vi "VFP Network Set Binding Attributes.vi"(9 "Access Type Strings":string[](array[string]), 10 "Ctl Ref Cluster":T2, 11 "attributes":T1) -> (3 "attributes out":T1)   [LabVIEW 2016]
uses:
  <resource>/dialog/variable/SCT Attributes.ctl
  <resource>/dialog/variable/FeaturePacks/Network/VFP Network ControlRef.ctl
  <resource>/dialog/variable/FeaturePacks/Utility/VFP Util Fetch Bool Control.vi
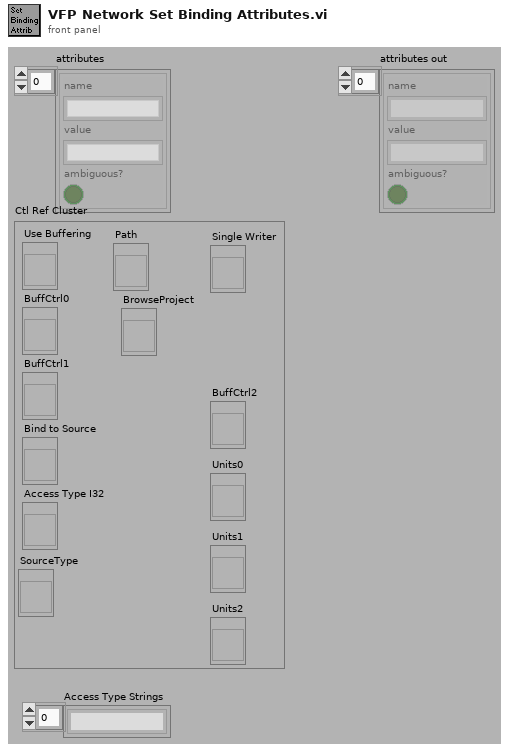
[diagram p1: front panel]
types:
  T1 = typedef "SCT Attributes.ctl" = cluster{"name":string, "value":string, "ambiguous?":bool}[]
  T2 = typedef "VFP Network ControlRef.ctl" = cluster{"Use Buffering":refnum<vi>, "BuffCtrl0":refnum<vi>, "BuffCtrl1":refnum<vi>, "Bind to Source":refnum<vi>, "Access Type I32":refnum<vi>, "Path":refnum<vi>, "BrowseProject":refnum<vi>, "Single Writer":refnum<vi>, "BuffCtrl2":refnum<vi>, "Units0":refnum<vi>, "Units1":refnum<vi>, "Units2":refnum<vi>, "SourceType":refnum<vi>}
  T3 = cluster{"name":string, "value":string, "ambiguous?":bool}
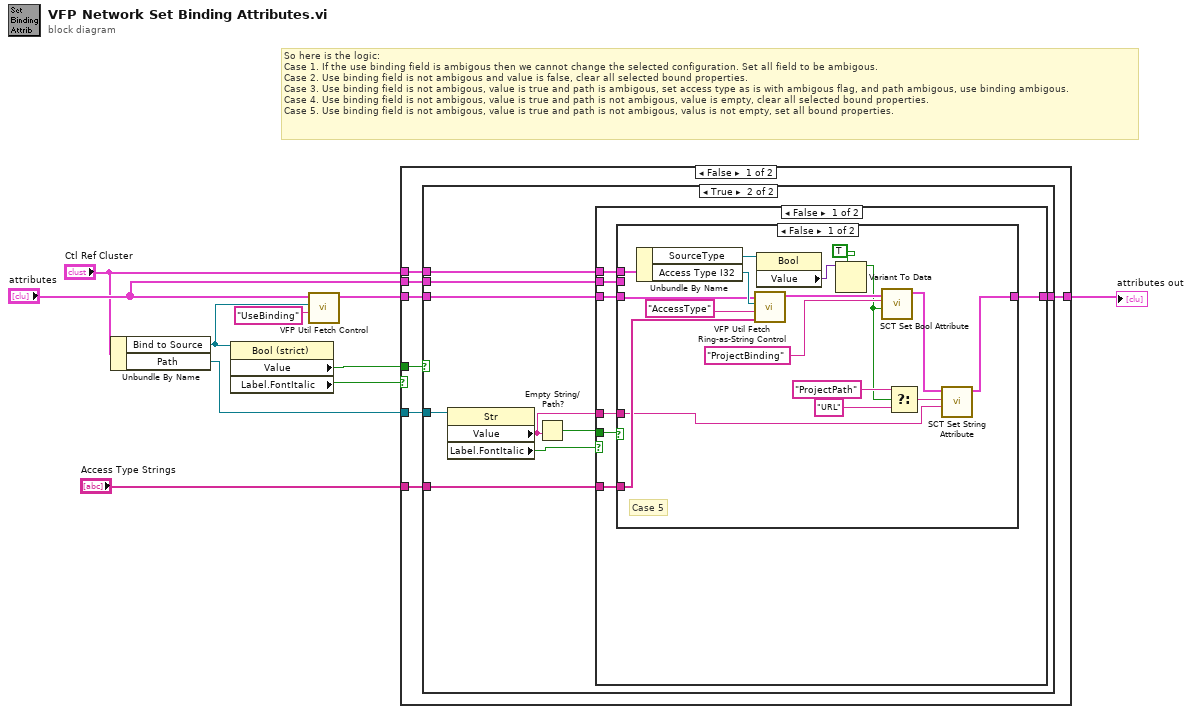
[diagram p0: block diagram]
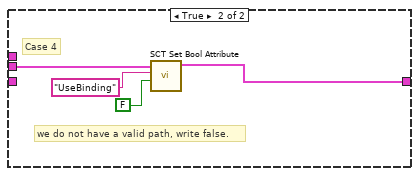
[diagram p3: hidden frame]
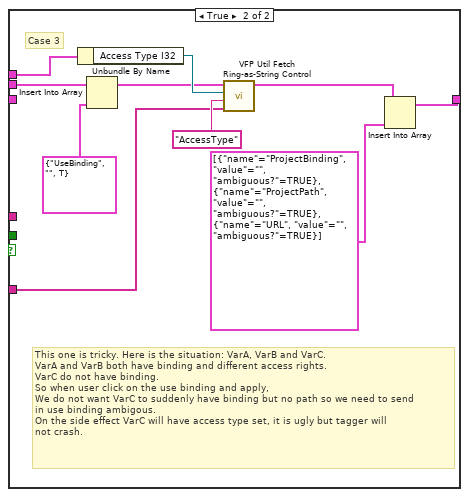
[diagram p4: hidden frame]
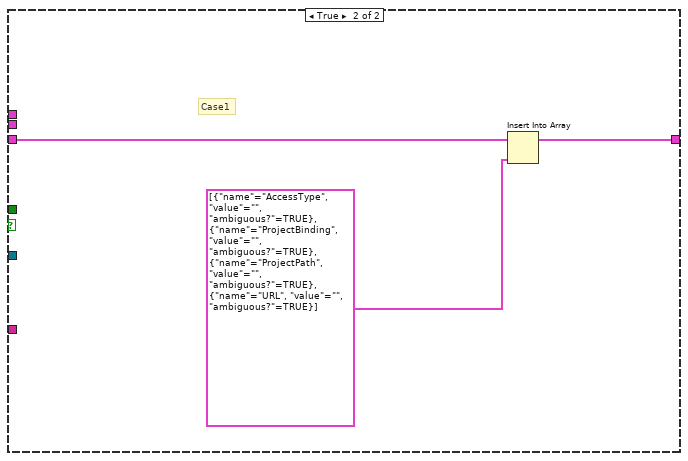
[diagram p5: hidden frame]
diagram:
  # "So here is the logic:\nCase 1. If the use binding field is ambigous then we cannot change the selected configuration. Set all field to be ambigous.\nCase 2. Use binding field is not ambigous and value is false, clear all selected bound properties.\nCase 3. Use binding field is not ambigous, value is true and path is ambigous, set access type as is with ambigous flag, and path ambigous, use binding ambigous.\nCase 4. Use binding field is not ambigous, value is true and path is not ambigous, value is empty, clear all selected bound properties.\nCase 5. Use binding field is not ambigous, value is true and path is not ambigous, valus is not empty, set all bound properties."
  n1 = Unbundle By Name("Ctl Ref Cluster") -> ("Bind to Source"=w2:refnum<vi>, "Path"=w1:refnum<vi>)
  n2 = property class="Bool (strict)"(reference=w2) -> ("Value"=w7:bool, "Label.FontItalic"=w4:bool)  [unwired: 1 in, 2 out]
  n3 = call-poly <resource>:"VFP Util Fetch Control.vi"("attribute name"="UseBinding", "control"=w2, "attributes"="attributes") -> ("attributes out"=w5:T1)  [unwired: 7 in, 1 out]
  n4 = case shown="False" w4 {
    tunnel: w5 -> [w16 w68]
    tunnel: [w14 w66] -> w6
    tunnel: w7 -> [w15 _]
    tunnel: "Ctl Ref Cluster" -> [w17 _]
    tunnel: "Access Type Strings" -> [w13 _]
    tunnel: "attributes" -> [w12 _]
    tunnel: w1 -> [w11 _]
    frame False {
      n5 = case shown="True" w15 {
        tunnel: w17 -> [_ w26]
        tunnel: w16 -> [w18 w27]
        tunnel: [w18 w24] -> w14
        tunnel: w13 -> [_ w25]
        tunnel: w12 -> [_ w23]
        tunnel: w11 -> [_ w19]
        frame False {
          # "Case 2. Binding is off."
        }
        frame True {
          n6 = property class="Str"(reference=w19) -> ("Value"=w20:string, "Label.FontItalic"=w22:bool)  [unwired: 1 in, 2 out]
          n7 = Empty String/Path?(string/path=w20) -> (empty?=w21:bool)
          n8 = case shown="False" w22 {
            tunnel: w27 -> [w33 _]
            tunnel: w26 -> [w31 w65]
            tunnel: w25 -> [w30 w62]
            tunnel: [w32 w59] -> w24
            tunnel: w21 -> [w34 _]
            tunnel: w20 -> [w29 _]
            tunnel: w23 -> [w28 w58]
            frame False {
              n9 = case shown="False" w34 {
                tunnel: w33 -> [w48 _]
                tunnel: [w36 w54] -> w32
                tunnel: w31 -> [w49 _]
                tunnel: w30 -> [w47 _]
                tunnel: w29 -> [w35 _]
                tunnel: w28 -> [_ w55]
                frame False {
                  # "Case 5"
                  n10 = Unbundle By Name(w49) -> ("SourceType"=w44:refnum<vi>, "Access Type I32"=w51:refnum<vi>)
                  n11 = call <resource>:"VFP Util Fetch Ring-as-String Control.vi"("Ring Strings"=w47, "attribute name"="AccessType" ("name"), "control"=w51, "attributes"=w48) -> ("attributes out"=w46:T1)  [unwired: 7 in]
                  n12 = property class="Bool"(reference=w44) -> ("Value"=w43:variant)  [unwired: 1 in, 2 out]
                  n13 = Variant To Data(type=TRUE, Variant=w43) -> (data=w38:bool)  [unwired: 1 in, 1 out]
                  n14 = call <resource>:"SCT Set Bool Attribute.vi"("value"=w38, "attribute name"="ProjectBinding", "attributes"=w46) -> ("attributes out"=w37:T1)  [unwired: 8 in]
                  n15 = Select(t="ProjectPath" ("attribute name"), s=w38, f="URL" ("name")) -> (s? t:f=w41:string)
                  n16 = call <resource>:"SCT Set String Attribute.vi"("value"=w35, "attribute name"=w41, "attributes"=w37) -> ("attributes out"=w36:T1)  [unwired: 8 in]
                }
                frame True {
                  # "we do not have a valid path, write false."
                  # "Case 4"
                  n17 = call <resource>:"SCT Set Bool Attribute.vi"("value"=FALSE, "attribute name"="UseBinding", "attributes"=w55) -> ("attributes out"=w54:T1)  [unwired: 8 in]
                }
              }
            }
            frame True {
              # "This one is tricky. Here is the situation: VarA, VarB and VarC.\nVarA and VarB both have binding and different access rights.\nVarC do not have binding.\nSo when user click on the use binding and apply,\nWe do not want VarC to suddenly have binding but no path so we need to send\nin use binding ambigous.\nOn the side effect VarC will have access type set, it is ugly but tagger will\nnot crash."
              # "Case 3"
              n18 = Unbundle By Name(w65) -> ("Access Type I32"=w64:refnum<vi>)
              n19 = Insert Into Array(array=w58, new element=T3 {"name"="UseBinding", "value"="", "ambiguous?"=TRUE} ("attribute")) -> (w56:T1)  [unwired: 1 in]
              n20 = call <resource>:"VFP Util Fetch Ring-as-String Control.vi"("Ring Strings"=w62, "attribute name"="AccessType" ("name"), "control"=w64, "attributes"=w56) -> ("attributes out"=w61:T1)  [unwired: 7 in]
              n21 = Insert Into Array(array=w61, new element=T1 [{"name"="ProjectBinding", "value"="", "ambiguous?"=TRUE}, {"name"="ProjectPath", "value"="", "ambiguous?"=TRUE}, {"name"="URL", "value"="", "ambiguous?"=TRUE}] ("attributes")) -> (w59:T1)  [unwired: 1 in]
            }
          }
        }
      }
    }
    frame True {
      # "Case1"
      n22 = Insert Into Array(array=w68, new element=T1 [{"name"="AccessType", "value"="", "ambiguous?"=TRUE}, {"name"="ProjectBinding", "value"="", "ambiguous?"=TRUE}, {"name"="ProjectPath", "value"="", "ambiguous?"=TRUE}, {"name"="URL", "value"="", "ambiguous?"=TRUE}] ("attributes")) -> (w66:T1)  [unwired: 1 in]
    }
  }
  "attributes out" <- w6
